vi "CloseVI.vi"(0 "VI Reference In":refnum<vi>, 11 "error in":errorcluster) -> (4 "VI Reference Out":refnum<vi>, 15 "error out":errorcluster)   [LabVIEW 2016, in "Drona.lvlib" / "VI.lvlib"]
doc: "Closes given VI by simulating Ctl + W."
uses:
  VI.lvlib
  KeyBoardSimulation/KeyBoardSimulationForTargetVI.vi
  Drona.lvlib
  KeyBoardSimulation/KeyboardSimulation.lvlib
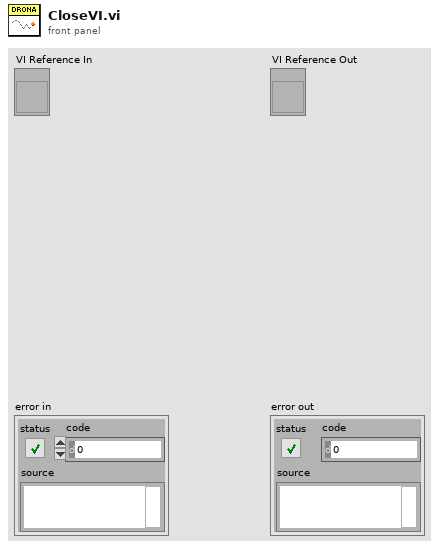
[diagram p1: front panel]
types:
  T1 = cluster{" Key":u8, "Action":enum16{"Press", "Up", "Down"}, "Delay (ms)":u32}[]
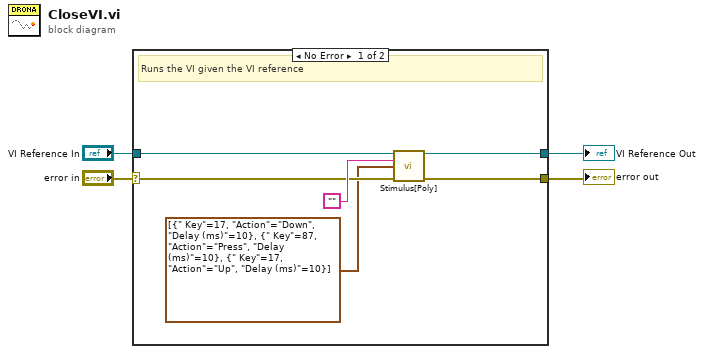
[diagram p0: block diagram]
diagram:
  n1 = case shown="No Error" "error in" {
    selector: "error in" -> [w9 w12]
    tunnel: "VI Reference In" -> [w6 w11]
    tunnel: [w7 w11] -> w2
    tunnel: [w8 w12] -> w1
    frame No Error {
      # "Runs the VI given the VI reference"
      n2 = call-poly "Stimulus[Poly].vi"("VI Reference In"=w6, "Control Path"="", "Key Array"=T1 [{" Key"=17, "Action"=enum."Down", "Delay (ms)"=10}, {" Key"=87, "Action"=enum."Press", "Delay (ms)"=10}, {" Key"=17, "Action"=enum."Up", "Delay (ms)"=10}], "error In"=w9) -> ("VI Reference Out"=w7:refnum<vi>, "error IO"=w8:errorcluster)  [unwired: 10 in]
    }
    frame Error {
    }
  }
  "error out" <- w1
  "VI Reference Out" <- w2
